vi "destroy.vi"(8 "error in (no error)":errorcluster, 11 "window":refnum<class "rywindow.lvclass">) -> (0 "error out":errorcluster)   [LabVIEW 2017, in "rywindow.lvclass"]
uses:
  rywindow.lvclass
  <vilib>/event_ctls.llb/usereventprio.ctl
  rywindow.lvclass/rywindow.ctl
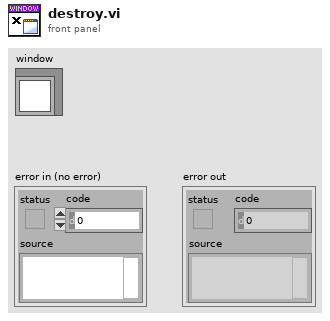
[diagram p1: front panel]
types:
  T1 = typedef "usereventprio.ctl" = enum32{"high priority", "normal priority"}
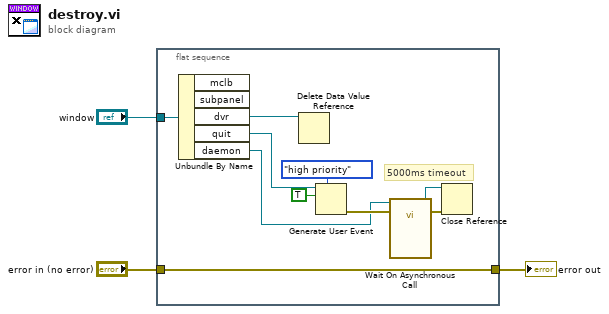
[diagram p0: block diagram]
diagram:
  n1 = flat-sequence {
    tunnel: "window" -> [w13]
    tunnel: [w4] -> w2
    tunnel: "error in (no error)" -> [w4]
    frame #0 {
      # "5000ms timeout"
      n2 = Unbundle By Name(w13) -> ("dvr"=w5:refnum<data-value>, "quit"=w12:refnum<user-event>, "daemon"=w8:refnum<vi>)  [unwired: 2 out]
      n3 = Delete Data Value Reference(data value reference=w5) -> ()  [unwired: 1 in, 2 out]
      n4 = Generate User Event(priority (normal)=usereventprio."high priority", user event=w12, event data cluster=TRUE ("event data")) -> (error out=w9:errorcluster)  [unwired: 1 in, 1 out]
      n5 = call-by-ref "Wait On Asynchronous Call"(reference=w8, error in=w9) -> (reference out=w6:refnum<vi>, error out=w7:errorcluster)  [unwired: 12 in]
      n6 = Close Reference(reference=w6, error in (no error)=w7) -> ()  [unwired: 1 out]
    }
  }
  "error out" <- w2
